vi "TextLog-Simple Log.vi"(7 "Message":string, 11 "error in":errorcluster) -> ()   [LabVIEW 2020]
uses:
  <vilib>/Utility/sysdir.llb/System Directory Type.ctl
  Error Handling VIs/Error-Library Action.ctl
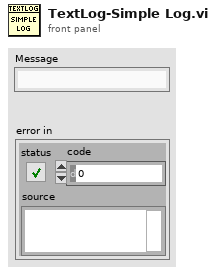
[diagram p1: front panel]
types:
  T1 = typedef "Error-Library Action.ctl" = enum16{"NONE", "Register", "Read"}
  T2 = typedef "System Directory Type.ctl" = i32
  T3 = typedef "Error Description.ctl" = cluster{"Code":i32, "Description":string, "Details":string}
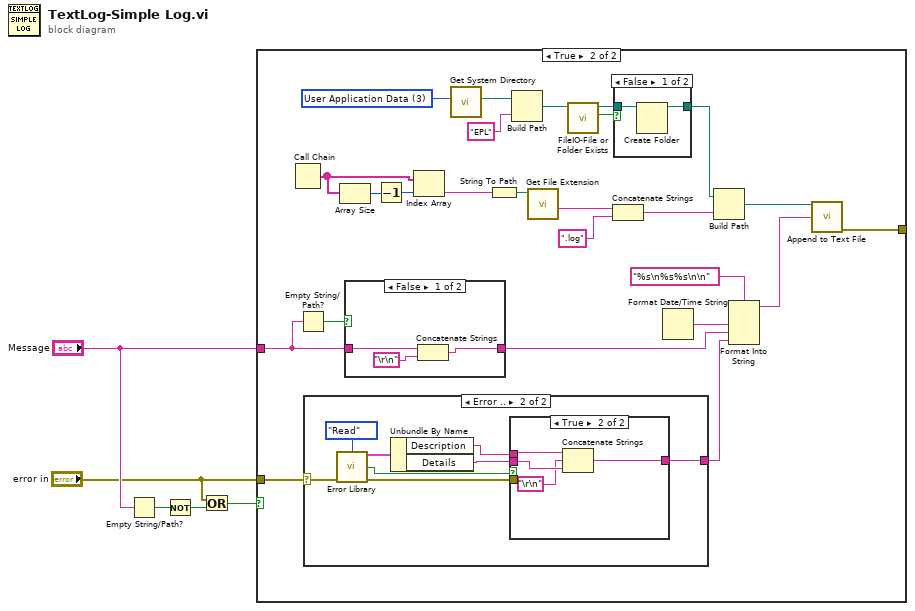
[diagram p0: block diagram]
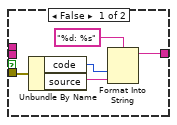
[diagram p6: hidden frame]
diagram:
  n1 = Empty String/Path?(string/path="Message") -> (empty?=w5:bool)
  n2 = Not(x=w5) -> (.not. x?=w4:bool)
  n3 = Or(x="error in", y=w4) -> (x .or. y?=w3:bool)
  n4 = case shown="True" w3 {
    tunnel: "Message" -> [_ w8]
    tunnel: "error in" -> [_ w14]
    tunnel: [_ w18] -> _
    frame False {
    }
    frame True {
      w28 = T2 3 items=["User Home", "User Desktop", "User Documents", "User Application Data", "User Preferences", "User Temporary", "Public Documents", "Public Application Data", "Public Preferences", "System Core Libraries", "System Installed Libraries", "Application Files", "Boot Volume Root"] ("system directory type")
      n5 = Call Chain() -> (call chain=w23:string[])
      n6 = Empty String/Path?(string/path=w8) -> (empty?=w7:bool)
      n7 = case shown="Error .." w14 {
        selector: w14 -> [_ w44]
        tunnel: [_ w45] -> w13
        frame No Error {
        }
        frame Error {
          n8 = call "Error Library.vi"("action"=Error-Library_Action."Read", "error in"=w44) -> ("Entry"=w39:T3, "found?"=w41:bool, "error thru"=w42:errorcluster)  [unwired: 11 in]
          n9 = Unbundle By Name(w39) -> ("Description"=w38:string, "Details"=w40:string)
          n10 = case shown="True" w41 {
            tunnel: w42 -> [w50 _]
            tunnel: w38 -> [_ w54]
            tunnel: w40 -> [_ w53]
            tunnel: [w49 w51] -> w45
            frame False {
              n11 = Unbundle By Name(w50) -> ("code"=w47:i32, "source"=w46:string)
              n12 = Format Into String(format string="%d: %s", w47, w46) -> (resulting string=w49:string)  [unwired: 2 in, 1 out]
            }
            frame True {
              n13 = Concatenate Strings(w54, "\r\n", w53) -> (w51:string)
            }
          }
        }
      }
      n14 = Array Size(array=w23) -> (size(s)=w22:i32)
      n15 = case shown="False" w7 {
        tunnel: w8 -> [w33 w34]
        tunnel: [w32 w34] -> w6
        frame False {
          n16 = Concatenate Strings(w33, "\r\n") -> (w32:string)
        }
        frame True {
        }
      }
      n17 = Decrement(x=w22) -> (x-1=w21:i32)
      n18 = Index Array(array=w23, index=w21) -> (element=w19:string)
      n19 = call <vilib>:"Get System Directory.vi"("system directory type"=w28) -> ("system directory"=w27:path)  [unwired: 10 in]
      n20 = String To Path(string=w19) -> (path=w20:path)
      n21 = Build Path(base path=w27, name or relative path="EPL") -> (appended path=w12:path)
      n22 = call <vilib>:"Get File Extension.vi"("file"=w20) -> ("filename without extension"=w25:string)  [unwired: 6 in, 4 out]
      n23 = call "FileIO-File or Folder Exists.vi"("path"=w12) -> ("Directory?"=w11:bool, "dup path"=w10:path)  [unwired: 7 in, 2 out]
      n24 = Concatenate Strings(w25, ".log" ("string")) -> (w29:string)
      n25 = case shown="False" w11 {
        tunnel: w10 -> [w36 w37]
        tunnel: [w35 w37] -> w9
        frame False {
          n26 = Create Folder(path (use dialog)=w36) -> (created path=w35:path)  [unwired: 2 in, 2 out]
        }
        frame True {
        }
      }
      n27 = Format Date/Time String() -> (date/time string=w16:string)  [unwired: 3 in]
      n28 = Build Path(base path=w9, name or relative path=w29) -> (appended path=w24:path)
      n29 = Format Into String(format string="%s\n%s%s\n\n", w16, w6, w13) -> (resulting string=w15:string)  [unwired: 2 in, 1 out]
      n30 = call "Append to Text File.vi"("file path"=w24, "text"=w15) -> ("error out"=w18:errorcluster)  [unwired: 12 in, 1 out]
    }
  }
